vi "tablet.vi"(11 "Shared_strings":string[][](array[string])) -> ()   [LabVIEW 2018]
uses:
  Global Variables.vi
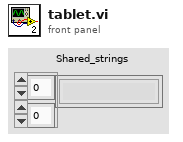
[diagram p1: front panel]
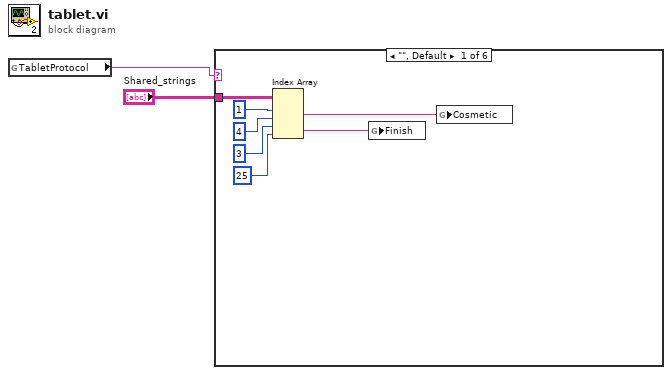
[diagram p0: block diagram]
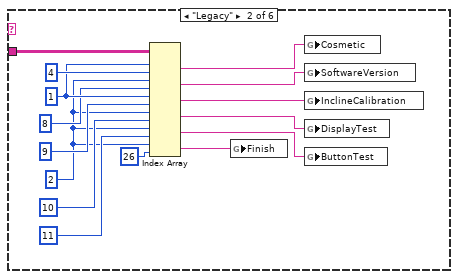
[diagram p2: hidden frame]
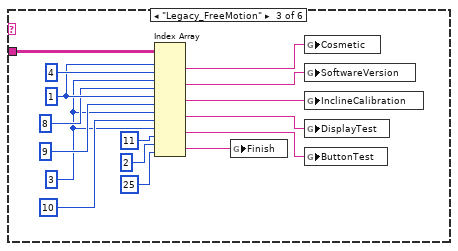
[diagram p3: hidden frame]
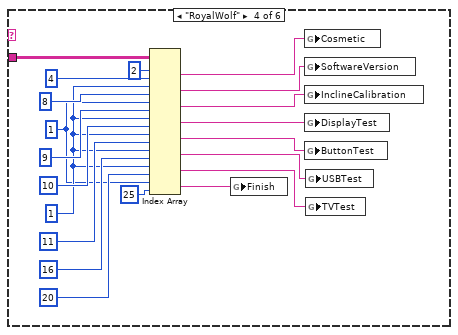
[diagram p4: hidden frame]
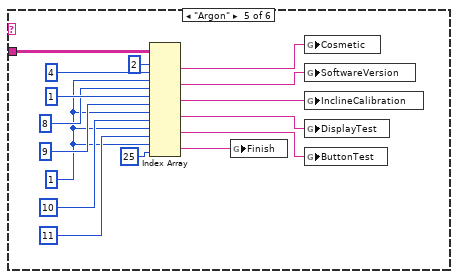
[diagram p5: hidden frame]
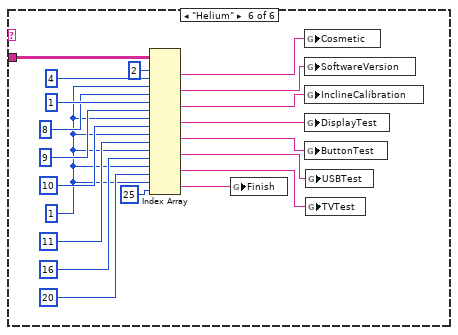
[diagram p6: hidden frame]
diagram:
  n1 = global read "Global Variables.vi" "TabletProtocol"() -> (w1:string)
  n2 = case shown="\"\", Default" w1 {
    tunnel: "Shared_strings" -> [w9 w23 w28 w50 w65 w81]
    frame "", Default {
      n3 = Index Array(array=w9, index (row) #1=1, index (col) #1=4, index (row) #2=3, index (col) #2=25) -> (element #1=w6:string, element #2=w5:string)
      n4 = global write "Global Variables.vi" "Finish"(w5) -> ()
      n5 = global write "Global Variables.vi" "Cosmetic"(w6) -> ()
    }
    frame "Legacy" {
      w11 = 2
      w21 = 1
      n6 = Index Array(array=w23, index (row) #1=w21, index (col) #1=4, index (row) #2=w11, index (col) #2=8, index (row) #3=w21, index (col) #3=9, index (row) #4=w11, index (col) #4=10, index (row) #5=w11, index (col) #5=11, index (row) #6=w11, index (col) #6=26) -> (element #1=w22:string, element #2=w17:string, element #3=w15:string, element #4=w16:string, element #5=w13:string, element #6=w10:string)
      n7 = global write "Global Variables.vi" "Finish"(w10) -> ()
      n8 = global write "Global Variables.vi" "Cosmetic"(w22) -> ()
      n9 = global write "Global Variables.vi" "SoftwareVersion"(w17) -> ()
      n10 = global write "Global Variables.vi" "InclineCalibration"(w15) -> ()
      n11 = global write "Global Variables.vi" "DisplayTest"(w16) -> ()
      n12 = global write "Global Variables.vi" "ButtonTest"(w13) -> ()
    }
    frame "Legacy_FreeMotion" {
      w31 = 3
      w38 = 1
      n13 = Index Array(array=w28, index (row) #1=w38, index (col) #1=4, index (row) #2=w31, index (col) #2=8, index (row) #3=w38, index (col) #3=9, index (row) #4=w31, index (col) #4=10, index (row) #5=w31, index (col) #5=11, index (row) #6=2, index (col) #6=25) -> (element #1=w39:string, element #2=w34:string, element #3=w32:string, element #4=w33:string, element #5=w29:string, element #6=w25:string)
      n14 = global write "Global Variables.vi" "Finish"(w25) -> ()
      n15 = global write "Global Variables.vi" "Cosmetic"(w39) -> ()
      n16 = global write "Global Variables.vi" "SoftwareVersion"(w34) -> ()
      n17 = global write "Global Variables.vi" "InclineCalibration"(w32) -> ()
      n18 = global write "Global Variables.vi" "DisplayTest"(w33) -> ()
      n19 = global write "Global Variables.vi" "ButtonTest"(w29) -> ()
    }
    frame "RoyalWolf" {
      w48 = 1
      w43 = 1
      n20 = Index Array(array=w50, index (row) #1=2 ("disabled index (row)"), index (col) #1=4, index (row) #2=w48, index (col) #2=8, index (row) #3=w43, index (col) #3=9, index (row) #4=w48, index (col) #4=10, index (row) #5=w48, index (col) #5=11, index (row) #6=w48, index (col) #6=16, index (row) #7=w48, index (col) #7=20, index (row) #8=w43, index (col) #8=25) -> (element #1=w59:string, element #2=w55:string, element #3=w53:string, element #4=w54:string, element #5=w51:string, element #6=w46:string, element #7=w45:string, element #8=w42:string)
      n21 = global write "Global Variables.vi" "Finish"(w42) -> ()
      n22 = global write "Global Variables.vi" "Cosmetic"(w59) -> ()
      n23 = global write "Global Variables.vi" "SoftwareVersion"(w55) -> ()
      n24 = global write "Global Variables.vi" "InclineCalibration"(w53) -> ()
      n25 = global write "Global Variables.vi" "DisplayTest"(w54) -> ()
      n26 = global write "Global Variables.vi" "ButtonTest"(w51) -> ()
      n27 = global write "Global Variables.vi" "USBTest"(w46) -> ()
      n28 = global write "Global Variables.vi" "TVTest"(w45) -> ()
    }
    frame "Argon" {
      w63 = 1
      n29 = Index Array(array=w65, index (row) #1=2 ("disabled index (row)"), index (col) #1=4, index (row) #2=w63, index (col) #2=8, index (row) #3=1, index (col) #3=9, index (row) #4=w63, index (col) #4=10, index (row) #5=w63, index (col) #5=11, index (row) #6=w63, index (col) #6=25) -> (element #1=w75:string, element #2=w70:string, element #3=w68:string, element #4=w69:string, element #5=w66:string, element #6=w62:string)
      n30 = global write "Global Variables.vi" "Finish"(w62) -> ()
      n31 = global write "Global Variables.vi" "Cosmetic"(w75) -> ()
      n32 = global write "Global Variables.vi" "SoftwareVersion"(w70) -> ()
      n33 = global write "Global Variables.vi" "InclineCalibration"(w68) -> ()
      n34 = global write "Global Variables.vi" "DisplayTest"(w69) -> ()
      n35 = global write "Global Variables.vi" "ButtonTest"(w66) -> ()
    }
    frame "Helium" {
      w78 = 1
      n36 = Index Array(array=w81, index (row) #1=2 ("disabled index (row)"), index (col) #1=4, index (row) #2=w78, index (col) #2=8, index (row) #3=1, index (col) #3=9, index (row) #4=w78, index (col) #4=10, index (row) #5=w78, index (col) #5=11, index (row) #6=w78, index (col) #6=16, index (row) #7=w78, index (col) #7=20, index (row) #8=w78, index (col) #8=25) -> (element #1=w95:string, element #2=w90:string, element #3=w88:string, element #4=w89:string, element #5=w86:string, element #6=w83:string, element #7=w82:string, element #8=w80:string)
      n37 = global write "Global Variables.vi" "Finish"(w80) -> ()
      n38 = global write "Global Variables.vi" "Cosmetic"(w95) -> ()
      n39 = global write "Global Variables.vi" "SoftwareVersion"(w90) -> ()
      n40 = global write "Global Variables.vi" "InclineCalibration"(w88) -> ()
      n41 = global write "Global Variables.vi" "DisplayTest"(w89) -> ()
      n42 = global write "Global Variables.vi" "ButtonTest"(w86) -> ()
      n43 = global write "Global Variables.vi" "USBTest"(w83) -> ()
      n44 = global write "Global Variables.vi" "TVTest"(w82) -> ()
    }
  }
